vi "Coursework working.vi"() -> ()   [LabVIEW 2014]
panel:
  in  "Close\nClose":bool
  in  "?":dbl(knob) scale=1000.0..100.0
  in  "?":dbl(knob) scale=1000.0..100.0
  in  "Reset":bool
  in  "First Location to Last":bool
  in  "Last Location to First":bool
  in  "?":bool
  out "?":cluster{"X":dbl[], "Y":dbl[]}[](graph)
  out "?":cluster{"Horizontal":dbl, dbl}[](graph)
  out "?":cluster{"Horizontal":dbl, dbl}[](graph)
  # "Instructions:\n\n1. Run the program\n2. Click the location of 10 destinations on the map\n3. Use the appropriate dials to speed up or speed down the simulation (program will not simulate unless a speed is chosen).\n4. If you would like a simulation choose one of the options:\n                            > From last location to first\n                            > From first location to last\n5. Click the reset button to clear the route and to start a new one"
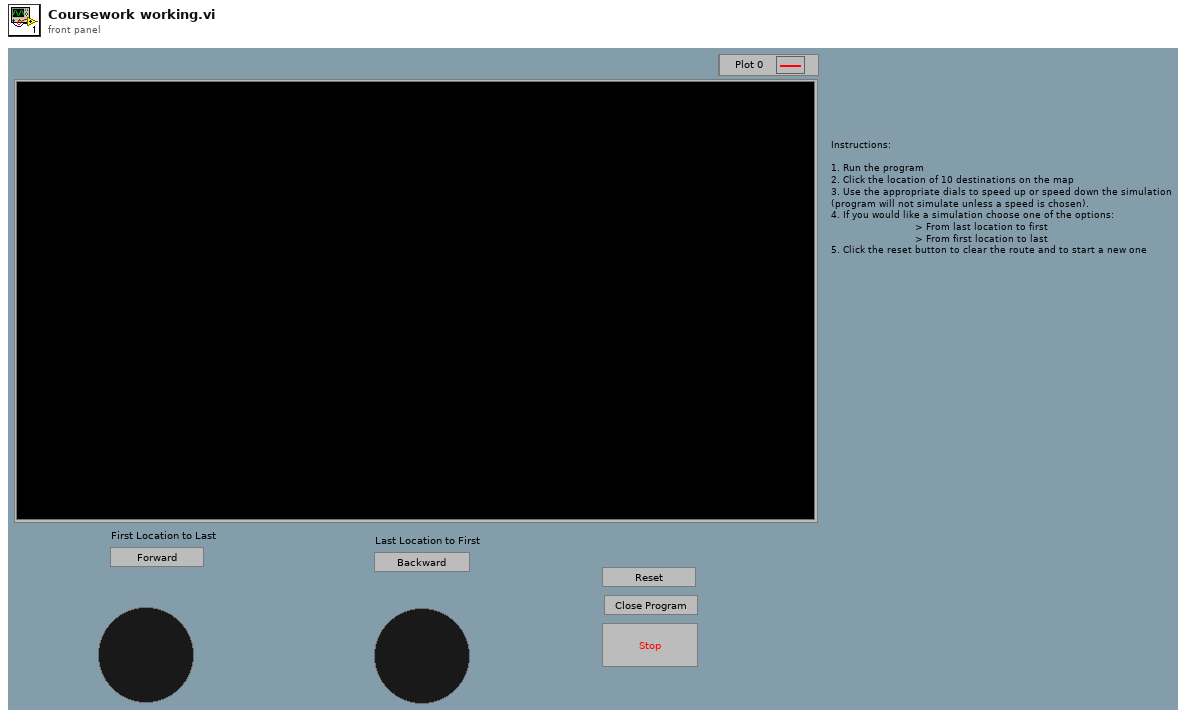
[diagram p1: front panel]
types:
  T1 = typedef "LVPoint32TypeDef.ctl" = cluster{"Horizontal":i32, "Vertical":i32}
  T2 = typedef "imagedata.ctl" = cluster{"image type":i32, "image depth":i32, "image":u8[], "mask":u8[], "colors":u32[], "Rectangle":cluster{"left":i16, "top":i16, "right":i16, "bottom":i16}}
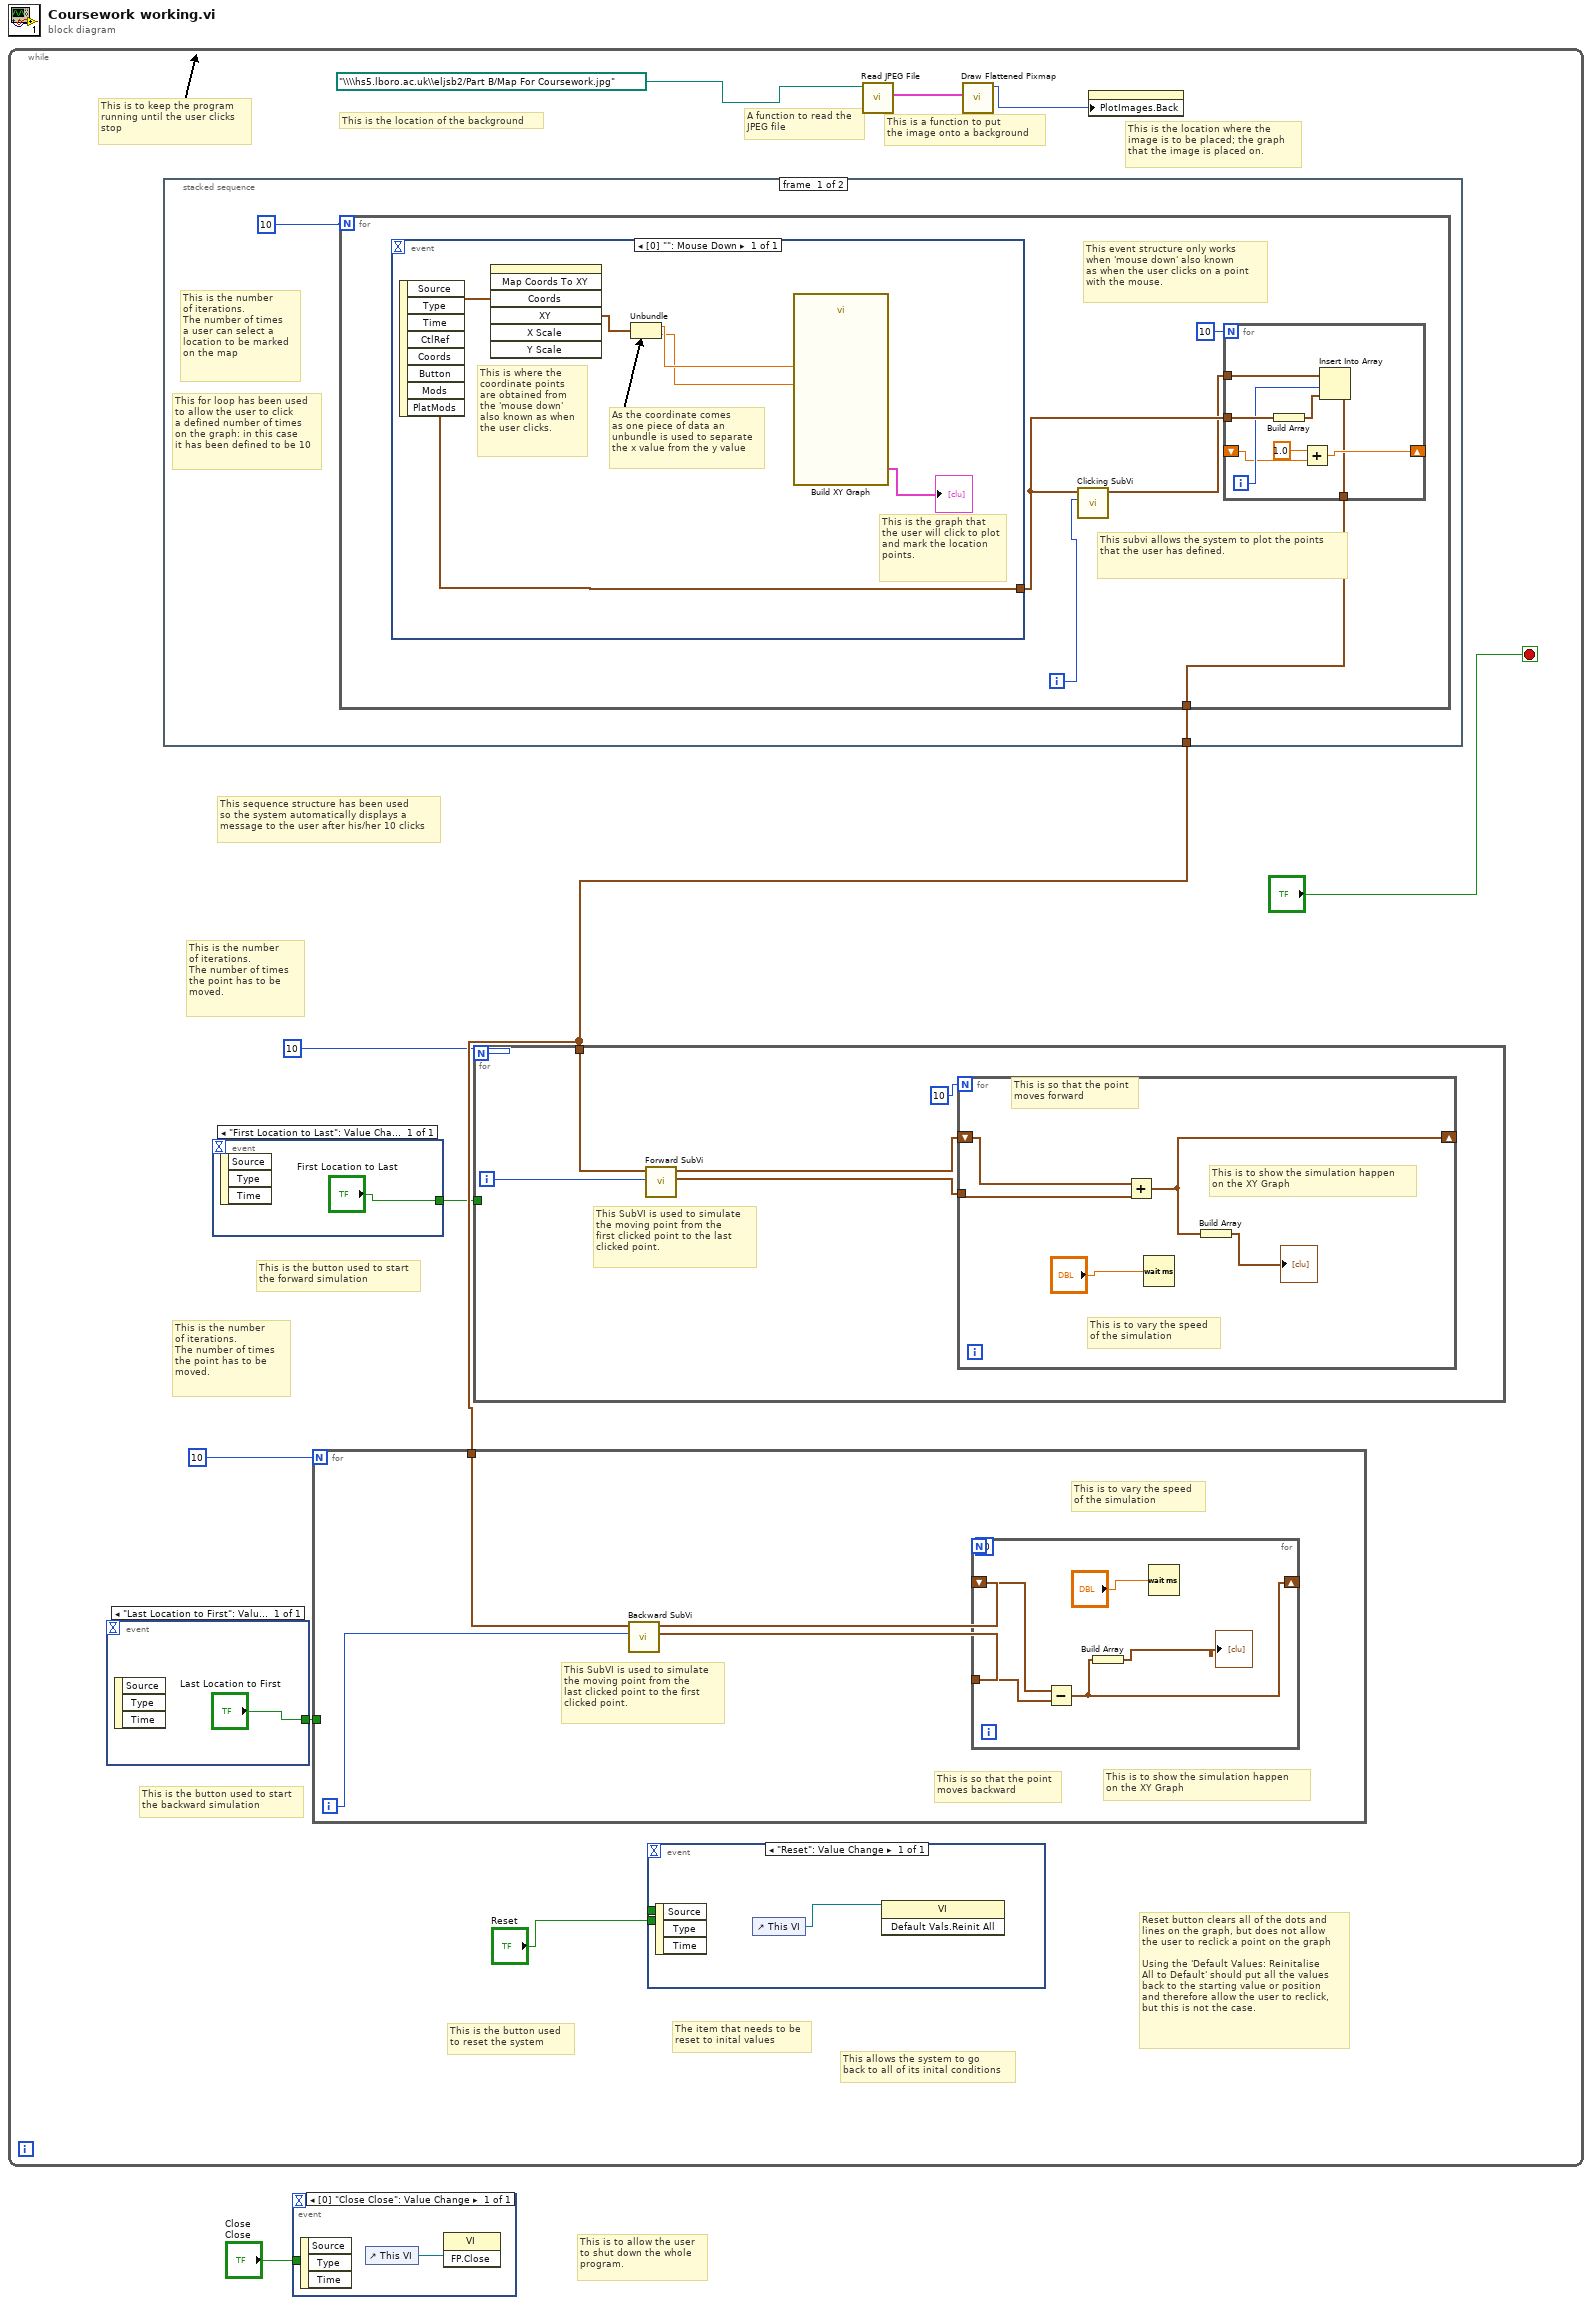
[diagram p0: block diagram]
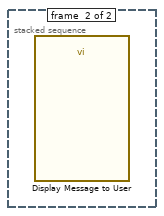
[diagram p2: hidden frame]
diagram:
  # "This is to allow the user \nto shut down the whole\nprogram."
  n1 = while {
    stop <- "?" stop-if-true
    # "Reset button clears all of the dots and \nlines on the graph, but does not allow \nthe user to reclick a point on the graph\n\nUsing the 'Default Values: Reinitalise \nAll to Default' should put all the values \nback to the starting value or position \nand therefore allow the user to reclick,\nbut this is not the case."
    # "This sequence structure has been used \nso the system automatically displays a \nmessage to the user after his/her 10 clicks"
    # "This is to keep the program \nrunning until the user clicks \nstop"
    # "The item that needs to be\nreset to inital values"
    # "This allows the system to go \nback to all of its inital conditions"
    # "This is the button used \nto reset the system"
    # "This is the button used to start\nthe backward simulation"
    # "This is the button used to start\nthe forward simulation"
    # "This is the number \nof iterations.\nThe number of times \nthe point has to be \nmoved."
    # "This is the number \nof iterations.\nThe number of times \nthe point has to be \nmoved."
    # "This is the location where the \nimage is to be placed; the graph \nthat the image is placed on."
    # "This is a function to put\nthe image onto a background"
    # "A function to read the\nJPEG file"
    # "This is the location of the background"
    n2 = event shown="[0] \"Last Location to First\": Value Change" {
      selector: _ -> [_]
      dyn-events: _ -> [_]
      timeout: _ -> [_]
      tunnel: ["Last Location to First"] -> w9
      event "Last Location to First": Value Change {
        n3 = event-data() -> ()  [unwired: 1 in, 3 out]
      }
    }
    n4 = stacked-sequence {
      tunnel: [w13 _] -> w10
      frame #0 {
        # "This for loop has been used\nto allow the user to click \na defined number of times\non the graph: in this case \nit has been defined to be 10"
        # "This is the number \nof iterations.\nThe number of times \na user can select a \nlocation to be marked\non the map"
        n5 = for {
          N: 10 -> [_]
          tunnel: [w14] -> w13
          i -> [w18]
          # "This event structure only works\nwhen 'mouse down' also known \nas when the user clicks on a point \nwith the mouse."
          # "This subvi allows the system to plot the points \nthat the user has defined."
          n6 = event shown="[0] \"\": Mouse Down" {
            selector: _ -> [_]
            dyn-events: _ -> [_]
            timeout: _ -> [_]
            tunnel: [w28] -> w16
            event Mouse Down {
              # "As the coordinate comes \nas one piece of data an \nunbundle is used to separate\nthe x value from the y value"
              # "This is where the\ncoordinate points \nare obtained from \nthe 'mouse down' \nalso known as when\nthe user clicks."
              # "This is the graph that the user will click to plot and mark the location points."
              n7 = event-data() -> ("Coords"=w28:T1)  [unwired: 1 in, 7 out]
              n8 = invoke class="XYGraph (strict)" method="Map Coords To XY"("Coords"=w28) -> ("XY"=w29:cluster{"X":dbl, "Y":dbl})  [unwired: 6 in, 6 out]
              n9 = Unbundle(w29) -> ("X"=w31:dbl, "Y"=w30:dbl)
              n10 = call "Build XY Graph"("Y Input"=w30, "X Input"=w31) -> ("XY Graph"=→"?":cluster{"X":dbl[], "Y":dbl[]}[])  [unwired: 8 in, 1 out]
            }
          }
          n11 = call "Clicking SubVi.vi"("Numeric"=w18, "Coords"=w16) -> ("Array"=w15:cluster{"Horizontal":i32, i32}[])  [unwired: 9 in]
          n12 = for {
            N: 10 -> [_]
            tunnel: w16 -> [w26]
            tunnel: w15 -> [w23]
            shift-right: [w21] -> _
            shift-left: _ -> [w22]
            tunnel: [w19] -> w14
            i -> [w24]
            n13 = Build Array(w26) -> (w25:T1[])
            n14 = Add(x=1.0, y=w22) -> (x+y=w21:dbl)
            n15 = Insert Into Array(array=w23, index=w24, new element=w25) -> (w19:cluster{"Horizontal":i32, i32}[])
          }
        }
      }
      frame #1 {
        n16 = call "Display Message to User"() -> ()  [unwired: 10 in, 2 out]
      }
    }
    n17 = event shown="[0] \"First Location to Last\": Value Change" {
      selector: _ -> [_]
      dyn-events: _ -> [_]
      timeout: _ -> [_]
      tunnel: ["First Location to Last"] -> w5
      event "First Location to Last": Value Change {
        n18 = event-data() -> ()  [unwired: 1 in, 3 out]
      }
    }
    n19 = for {
      N: 10 -> [_]
      tunnel: w10 -> [w46]
      tunnel: w9 -> [_]
      i -> [w47]
      # "This is so that the point\nmoves backward"
      # "This is to show the simulation happen \non the XY Graph"
      # "This is to vary the speed \nof the simulation"
      # "This SubVI is used to simulate \nthe moving point from the \nlast clicked point to the first \nclicked point."
      n20 = call "Backward SubVi.vi"("Numeric"=w47, "Array"=w46) -> ("Cluster 2"=w50:cluster{"Horizontal":dbl, dbl}, "Cluster"=w48:cluster{"Horizontal":i32, i32})  [unwired: 8 in]
      n21 = for {
        N: 10 -> [_]
        tunnel: w50 -> [w52]
        shift-right: [w55] -> _
        shift-left: w48 -> [w53]
        n22 = Subtract(x=w53, y=w52) -> (x-y=w55:cluster{"Horizontal":dbl, dbl})
        n23 = Build Array(w55) -> (→"?":cluster{"Horizontal":dbl, dbl}[])
        n24 = Wait (ms)(milliseconds to wait="?") -> ()  [unwired: 1 out]
      }
    }
    n25 = for {
      N: 10 -> [_]
      tunnel: w10 -> [w34]
      tunnel: w5 -> [_]
      i -> [w37]
      # "This SubVI is used to simulate \nthe moving point from the \nfirst clicked point to the last \nclicked point."
      n26 = call "Forward SubVi.vi"("Numeric"=w37, "Array"=w34) -> ("Cluster 2"=w36:cluster{"Horizontal":dbl, dbl}, "Cluster"=w35:cluster{"Horizontal":i32, i32})  [unwired: 8 in]
      n27 = for {
        N: 10 -> [_]
        tunnel: w36 -> [w42]
        shift-right: [w39] -> _
        shift-left: w35 -> [w41]
        # "This is so that the point\nmoves forward"
        # "This is to show the simulation happen \non the XY Graph"
        # "This is to vary the speed \nof the simulation"
        n28 = Add(x=w41, y=w42) -> (x+y=w39:cluster{"Horizontal":dbl, dbl})
        n29 = Wait (ms)(milliseconds to wait="?") -> ()  [unwired: 1 out]
        n30 = Build Array(w39) -> (→"?":cluster{"Horizontal":dbl, dbl}[])
      }
    }
    n31 = event shown="[0] \"Reset\": Value Change" {
      selector: _ -> [_]
      dyn-events: _ -> [_]
      timeout: _ -> [_]
      tunnel: [w43] -> _
      tunnel: "Reset" -> [w43]
      event "Reset": Value Change {
        n32 = event-data() -> ()  [unwired: 1 in, 3 out]
        n33 = control-ref of="This VI"() -> (w44:refnum<vi>)
        n34 = invoke class="VI" method="Default Vals.Reinit All"(reference=w44) -> ()  [unwired: 2 in, 3 out]
      }
    }
    n35 = call <vilib>:"Read JPEG File.vi"("path to JPEG file"=path "\\\\hs5.lboro.ac.uk\\eljsb2/Part B/Map For Coursework.jpg" ("Path")) -> ("image data"=w3:T2)  [unwired: 8 in, 2 out]
    n36 = call <vilib>:"Draw Flattened Pixmap.vi"("image data"=w3) -> ("new picture"=w4:picture)  [unwired: 8 in]
    n37 = property class="XYGraph (strict)"("PlotImages.Back"=w4) -> ()  [unwired: 2 in, 2 out]
  }
  n38 = event shown="[0] \"Close Close\": Value Change" {
    selector: _ -> [_]
    dyn-events: _ -> [_]
    timeout: _ -> [_]
    tunnel: "Close\nClose" -> [_]
    event "Close\nClose": Value Change {
      n39 = event-data() -> ()  [unwired: 1 in, 3 out]
      n40 = control-ref of="This VI"() -> (w56:refnum<vi>)
      n41 = invoke class="VI" method="FP.Close"(reference=w56) -> ()  [unwired: 2 in, 3 out]
    }
  }
